vi "createBoosterValveGainFrame.vi"(8 "error in (no error)":errorcluster, 9 "TriggerIRQ":bool, 10 "WaitForTrigger":bool, 11 "FAILC in":refnum<class "FAILC.lvclass">) -> (0 "error out":errorcluster, 2 "TxFrame":T1 {"Data" format="%02x"}, 3 "FAILC out":refnum<class "FAILC.lvclass">)   [LabVIEW 2016, in "RTFAILC.lvlib" / "FAILC.lvclass"]
uses:
  FAILC.lvclass
  D:/Code/Common_RT_ILC/ILC/ILC.lvclass
  Common_RT_Modbus/DataTypes/TxFrame.ctl
  Common_RT_Modbus/DynamicFrameBuilder/DynamicFrameBuilder.lvclass
  FAILC.lvclass/FAILC.ctl
  Common_RT_ILC/ILC/ILC.lvclass/ILC.ctl
  Common_RT_ILC/ILC/ILC.lvclass
  Common_RT_Modbus/RTModbus.lvlib
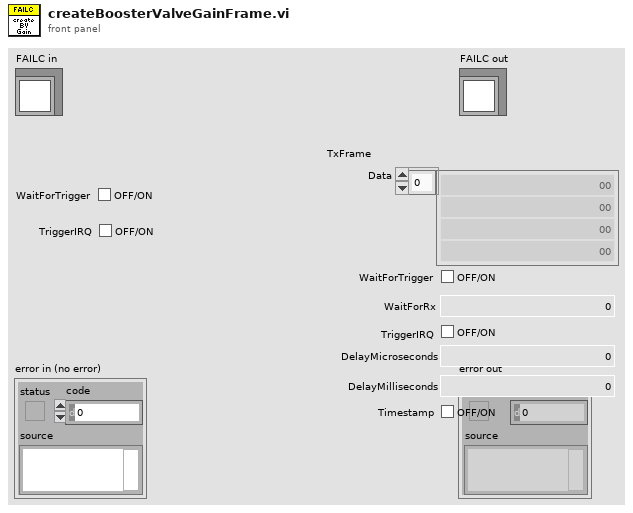
[diagram p1: front panel]
types:
  T1 = typedef "RTModbus.lvlib/TxFrame.ctl" = cluster{"Data":u8[], "WaitForTrigger":bool, "WaitForRx":u16, "TriggerIRQ":bool, "DelayMicroseconds":u16, "DelayMilliseconds":u16, "Timestamp":bool}
  T2 = typedef "RTILC.lvlib/ILCData.ctl" = cluster{"Constants":T3, "Command":T4, "Telemetry":T6, "Responses":T7, "Timings":T9}
  T3 = typedef "RTILC.lvlib/ILCConstants.ctl" = cluster{"Subnet":u8, "Address":u8}
  T4 = typedef "RTILC.lvlib/ILCCommand.ctl" = cluster{"ILCMode":u16, "TemporaryAddress":u8, "ADCScanRate":T5, "ADCChannel":u8, "ADCOffset":sgl, "ADCSensitivity":sgl}
  T5 = typedef "RTILC.lvlib/ILCScanRates.ctl" = u8
  T6 = typedef "RTILC.lvlib/ILCTelemetry.ctl" = cluster{"UniqueID":u64, "FirmwareType":u8, "NetworkNodeType":u8, "ILCOption":u8, "NetworkNodeOption":u8, "MajorRevision":u8, "MinorRevision":u8, "FirmwareName":string, "ILCMode":u16, "MajorFault":bool, "MinorFault":bool, "FaultOverride":bool, "UniqueIDCRCMismatch":bool, "AppTypeNodeTypeMismatch":bool, "AppMissing":bool, "AppCRCMismatch":bool, "TEDSNotFound":bool, "TEDS1Mismatch":bool, "TEDS2Mismatch":bool, "WatchdogResetDetected":bool, "BrownoutDetected":bool, "EventTrapResetDetected":bool, "TemporaryAddress":u8, "ADCScanRate":T5, "DAC1":u16, "DAC2":u16, "DAC3":u16, "DAC4":u16, "MainADCCalibrationK":sgl[], "MainSensorOffset":sgl[], "MainSensorSensitivity":sgl[], "BackupADCCalibrationK":sgl[], "BackupSensorOffset":sgl[], "BackupSensorSensitivity":sgl[]}
  T7 = typedef "RTILC.lvlib/ILCResponses.ctl" = cluster{"ReportServerID":T8, "ReportServerStatus":T8, "ILCMode":T8, "SetTemporaryAddress":T8, "Reset":T8, "ADCScanRate":T8, "ADCOffsetSensitivity":T8, "ReadDAC":T8, "ReadCalibration":T8}
  T8 = typedef "RTModbus.lvlib/ExceptionCodes.ctl" = u16
  T9 = typedef "RTILC.lvlib/ILCTimings.ctl" = cluster{"ADCOffsetSensitivity":u32, "ADCScanRate":u32, "ILCMode":u32, "ReadCalibration":u32, "ReportServerID":u32, "ReportServerStatus":u32, "Reset":u32, "SetTemporaryAddress":u32}
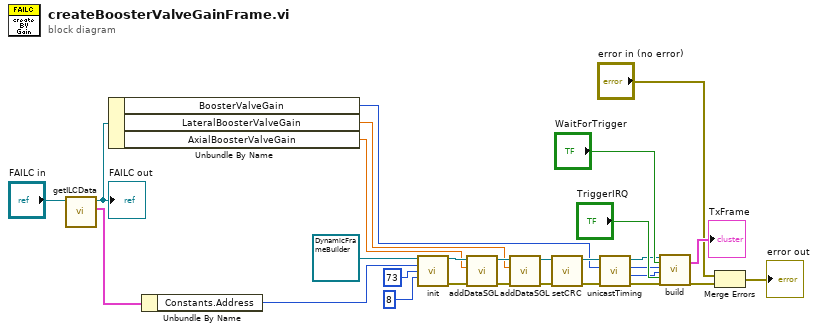
[diagram p0: block diagram]
diagram:
  n1 = call "getILCData.vi"("ILC in"="FAILC in") -> ("ILCData"=w26:T2, "ILC out"=w6:refnum<class "FAILC.lvclass">)  [unwired: 9 in]
  "FAILC out" <- w6
  n2 = Unbundle By Name(w6) -> ("BoosterValveGain"=w5:u32, "LateralBoosterValveGain"=w3:sgl, "AxialBoosterValveGain"=w4:sgl)
  n3 = Unbundle By Name(w26) -> ("Constants.Address"=w25:u8)
  n4 = call "init.vi"("DynamicFrameBuilder in"=refnum<class "DynamicFrameBuilder.lvclass"> refnum ("RTModbus.lvlib:DynamicFrameBuilder.lvclass"), "Address"=w25, "Function"=u8 73, "DataSize"=8) -> ("DynamicFrameBuilder out"=w16:refnum<class "DynamicFrameBuilder.lvclass">, "error out"=w22:errorcluster)  [unwired: 10 in]
  n5 = call "addDataSGL.vi"("error in (no error)"=w22, "Data"=w4, "DynamicFrameBuilder in"=w16) -> ("error out"=w21:errorcluster, "DynamicFrameBuilder out"=w17:refnum<class "DynamicFrameBuilder.lvclass">)  [unwired: 7 in]
  n6 = call "addDataSGL.vi"("error in (no error)"=w21, "Data"=w3, "DynamicFrameBuilder in"=w17) -> ("error out"=w1:errorcluster, "DynamicFrameBuilder out"=w2:refnum<class "DynamicFrameBuilder.lvclass">)  [unwired: 7 in]
  n7 = call "setCRC.vi"("error in (no error)"=w1, "DynamicFrameBuilder in"=w2) -> ("error out"=w9:errorcluster, "DynamicFrameBuilder out"=w12:refnum<class "DynamicFrameBuilder.lvclass">)  [unwired: 8 in]
  n8 = call "unicastTiming.vi"("error in (no error)"=w9, "Latency in"=w5, "DynamicFrameBuilder in"=w12) -> ("error out"=w10:errorcluster, "WaitForRxTimeout"=w7:u16, "Latency out"=w8:u32, "DynamicFrameBuilder out"=w11:refnum<class "DynamicFrameBuilder.lvclass">)  [unwired: 5 in]
  n9 = call "build.vi"("DynamicFrameBuilder in"=w11, "WaitForTrigger"="WaitForTrigger", "Latency"=w8, "WaitForRxTimeout"=w7, "TriggerIRQ"="TriggerIRQ", "error in (no error)"=w10) -> ("TxFrame"=→"TxFrame":T1, "error out"=w14:errorcluster)  [unwired: 11 in, 1 out]
  n10 = Merge Errors("error in (no error)", w14) -> (→"error out":errorcluster)
